vi "Switch Control.vi"(8 "error in (no error)":errorcluster, 10 "Finger Number":dbl=1.0 min=1.0 max=12.0 step=1.0 format="%0#2_2g", 11 "VISA Refnum in":refnum<visa-resource-name>) -> ()   [LabVIEW 2016]
uses:
  <vilib>/Instr/_visa.llb/VISA Configure Serial Port (Instr).vi
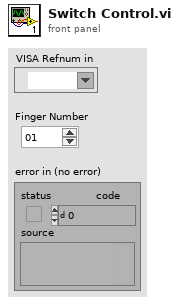
[diagram p1: front panel]
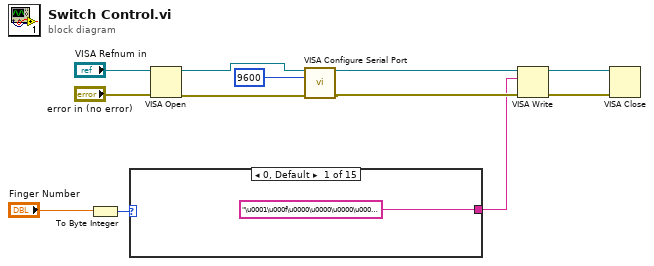
[diagram p0: block diagram]
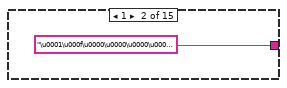
[diagram p2: hidden frame]
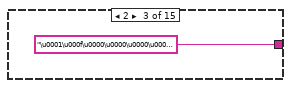
[diagram p3: hidden frame]
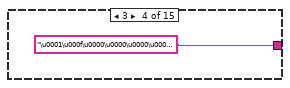
[diagram p4: hidden frame]
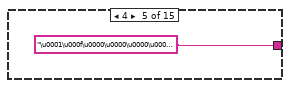
[diagram p5: hidden frame]
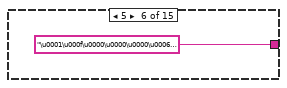
[diagram p6: hidden frame]
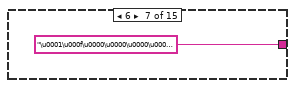
[diagram p7: hidden frame]
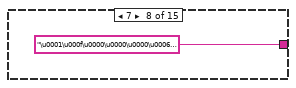
[diagram p8: hidden frame]
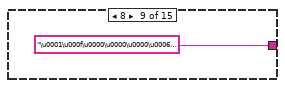
[diagram p9: hidden frame]
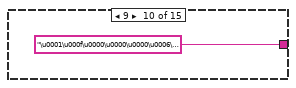
[diagram p10: hidden frame]
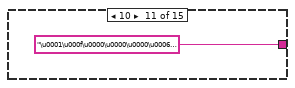
[diagram p11: hidden frame]
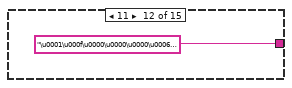
[diagram p12: hidden frame]
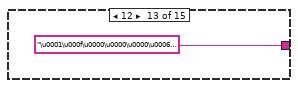
[diagram p13: hidden frame]
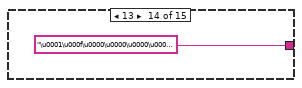
[diagram p14: hidden frame]
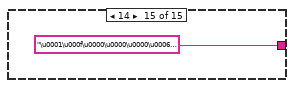
[diagram p15: hidden frame]
diagram:
  n1 = To Byte Integer(number="Finger Number") -> (8bit integer=w9:i8)
  n2 = case shown="0, Default" w9 {
    tunnel: ["\u0001\u000f\u0000\u0000\u0000\u0006\u0001\u0000ŸV" "\u0001\u000f\u0000\u0000\u0000\u0006\u0001\u0001^–" "\u0001\u000f\u0000\u0000\u0000\u0006\u0001\u0002\u001e—" "\u0001\u000f\u0000\u0000\u0000\u0006\u0001\u0004ž•" "\u0001\u000f\u0000\u0000\u0000\u0006\u0001\b" "\u0001\u000f\u0000\u0000\u0000\u0006\u0001\u0010žš" "\u0001\u000f\u0000\u0000\u0000\u0006\u0001 žŽ" "\u0001\u000f\u0000\u0000\u0000\u0006\u0001?ßF" "\u0001\u000f\u0000\u0000\u0000\u0006\u0001\u001fޞ" "\u0001\u000f\u0000\u0000\u0000\u0006\u0001/ފ" "\u0001\u000f\u0000\u0000\u0000\u0006\u00017ހ" "\u0001\u000f\u0000\u0000\u0000\u0006\u0001;ޅ" "\u0001\u000f\u0000\u0000\u0000\u0006\u0001=^‡" "\u0001\u000f\u0000\u0000\u0000\u0006\u0001>\u001e†" "\u0001\u000f\u0000\u0000\u0000\u0006\u0001\u0007ޔ"] -> w1
    frame 0, Default {
    }
    frame 1 {
    }
    frame 2 {
    }
    frame 3 {
    }
    frame 4 {
    }
    frame 5 {
    }
    frame 6 {
    }
    frame 7 {
    }
    frame 8 {
    }
    frame 9 {
    }
    frame 10 {
    }
    frame 11 {
    }
    frame 12 {
    }
    frame 13 {
    }
    frame 14 {
    }
  }
  n3 = VISA Open(error in (no error)="error in (no error)", VISA resource name="VISA Refnum in") -> (VISA resource name=w7:refnum<visa-resource-name>, error out=w8:errorcluster)  [unwired: 3 in]
  n4 = call-poly "VISA Configure Serial Port"("VISA resource name"=w7, "baud rate (9600)"=u32 9600, "error in (no error)"=w8) -> ("VISA resource name out"=w11:refnum<visa-resource-name>, "error out"=w12:errorcluster)  [unwired: 11 in]
  n5 = VISA Write(VISA resource name=w11, write buffer=w1, error in (no error)=w12) -> (VISA resource name out=w3:refnum<visa-resource-name>, error out=w4:errorcluster)  [unwired: 1 out]
  n6 = VISA Close(VISA resource name=w3, error in (no error)=w4) -> ()  [unwired: 1 out]
